vi "I2.vi"() -> ()   [LabVIEW 2020]
uses:
  <vilib>/Analysis/Matrix/Datatypes/RealMatrix.ctl
  <vilib>/Platform/TimedLoop/XDataNode/timing_clust.ctl
  <vilib>/Platform/TimedLoop/XDataNode/nitl_modes.ctl
  <vilib>/Platform/TimedLoop/XDataNode/wakeup.ctl
  <vilib>/Analysis/baseanly.llb/Real Dot Product.vi
  <vilib>/MakerHub/LINX/Public/Peripherals/PWM/PWM Set Duty Cycle 1 Chan.vi
  <vilib>/MakerHub/LINX/Public/Peripherals/Analog/Analog Read 1 Chan.vi
  <vilib>/MakerHub/LINX/Public/Peripherals/Analog/Analog Read N Chans.vi
  <vilib>/MakerHub/LINX/Private/Local IO/LinxAnalogRead.vi
  <vilib>/MakerHub/LINX/Public/Utilities/Check Channel.vi
  <vilib>/MakerHub/LINX/Public/Utilities/Open Serial.vi
  <vilib>/MakerHub/LINX/Public/Peripherals/PWM/PWM Set Duty Cycle N Chans.vi
  <vilib>/MakerHub/LINX/Private/Utilties/Generate Error.vi
  <vilib>/Analysis/polynomials.llb/Create Polynomial From Roots (CDB).vi
  <vilib>/platform/TimedLoop/XDataNode/XDataNode.xnode
  <vilib>/MakerHub/LINX/LMH-LINX.lvlib
  <vilib>/Platform/TimedLoop/XDataNode/XDNodeRunTimeDep.lvlib
  <vilib>/Analysis/NI_AALPro.lvlib
  <vilib>/Analysis/NI_AALBase.lvlib
  <vilib>/Analysis/Matrix/NI_Matrix.lvlib
panel:
  in  "file path (use dialog)":path
  out "corriente":dbl
  out "A":T1
  out "Regresor":dbl[](array[numeric])
  out "Pd(Z)":dbl[](array[numeric])
  out "p/q":dbl[](array[numeric]) format="%.4f"
  out "Theta":dbl[](array[numeric])
  in  "Parametros":T2={"Lambda"=0.987, "Alfa"=10000.0, "nb"=2, "d"=2, "na"=2, "b0? "=FALSE}
  in  "Pnd":cdb[](array[numeric])=[0.1+0.0i, 0.1+0.0i, 0.1+0.0i, 0.1+0.0i]
  in  "ts(s)":dbl=100.0
  in  "Tm":dbl=1.0
  in  "Mp(%)":dbl=5.0
  in  "Setpoint":dbl
  out "u(k)":dbl
  out "Temperatura":dbl
  out "x/y":dbl
  in  "stop":bool
  in  "Serial Port":refnum<visa-resource-name>="N/A"
  out "?":cluster{"Temperatura":dbl, dbl, "u(k)":dbl}(graph)
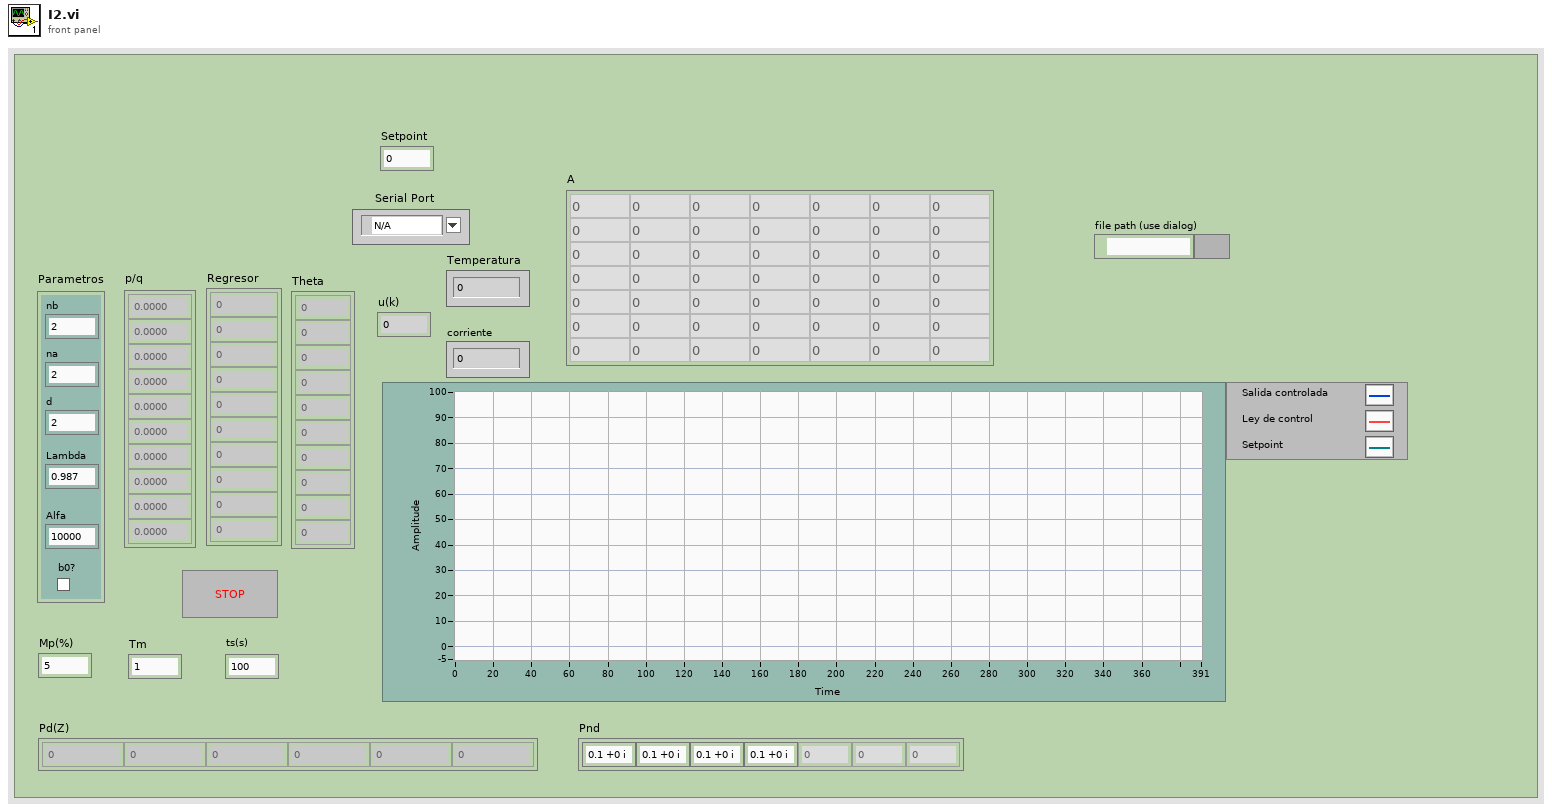
[diagram p1: front panel]
types:
  T1 = typedef "NI_Matrix.lvlib/RealMatrix.ctl" = dbl[][]
  T2 = cluster{"Lambda":dbl, "Alfa":dbl, "nb":u8, "d":u8, "na":u8, "b0? ":bool}
  T3 = enum16{"open", "replace", "create", "open or create", "replace or create", "replace or create with confirmation"}
  T4 = typedef "LMH-LINX.lvlib/LINX Ref.ctl" = cluster{"IO":T5, "Interface":T6, "LINX Device Config":T7}
  T5 = typedef "LMH-LINX.lvlib/Platform.ctl" = enum16{"Remote", "Local"}
  T6 = typedef "LMH-LINX.lvlib/Interface.ctl" = enum16{"Serial", "TCP"}
  T7 = typedef "LMH-LINX.lvlib/Device.lvlib/LINX Device Config.ctl" = cluster{"Interface":T6, "COM Port":refnum<visa-resource-name>, "TCP Configuration":T8, "Device Family":u8, "Device ID":u8, "Device Name":string, "TCP Ref":refnum<k5>, "Channels":T9}
  T8 = typedef "LMH-LINX.lvlib/Device.lvlib/TCP Config.ctl" = cluster{"IP Address":string, "Port":u16}
  T9 = typedef "LMH-LINX.lvlib/Channels.ctl" = cluster{"DI":u8[], "DO":u8[], "AI":u8[], "AO":u8[], "PWM":u8[], "QE":u8[], "UART":u8[], "I2C 2":u8[], "SPI":u8[], "CAN":u8[], "Servo":u8[], "AI Ref (V)":dbl, "AI Resolution (Bits)":u8, "AO Ref (V)":dbl, "AO Resolution (Bits)":u8}
  T10 = typedef "XDNodeRunTimeDep.lvlib/timing_clust.ctl" = cluster{"Expected End [f-1]":u64, "Actual End [f-1]":u64, "Finished Late? [f-1]":bool, "Expected End [i-1]":u64, "Actual End [i-1]":u64, "Finished Late? [i-1]":bool, "Expected Start [i]":u64, "Actual Start [i]":u64, "Expected Start [f]":u64, "Actual Start [f]":u64, "Source Name":string, "Structure Name":string, "Period":i64, "Deadline":i64, "Offset":i64, "Start":i64, "Priority":i32, "Timeout":i32, "Mode":T11, "Wakeup Reason":T12, "Error":errorcluster, "Source Type":string, "Secondary Source Type":string, "Global End Time":u64, "Global Start Time":u64, "Frame Duration":u64, "Iteration Duration":u64, "Assigned CPU":i32, "I/O Scan Engine Mode":u32}
  T11 = typedef "XDNodeRunTimeDep.lvlib/nitl_modes.ctl" = enum32{"No Change", "Process missed periods, maintain original phase", "Discard missed periods, maintain original phase", "Process missed periods, ignore original phase", "Discard missed periods, ignore original phase"}
  T12 = typedef "XDNodeRunTimeDep.lvlib/wakeup.ctl" = enum32{"Normal", "Aborted", "Asynchronous wakeup", "Timing source error", "Timed loop error", "Timeout"}
  T13 = cluster{"Temperatura":dbl, "u(k)":dbl, "Setpoint":dbl}
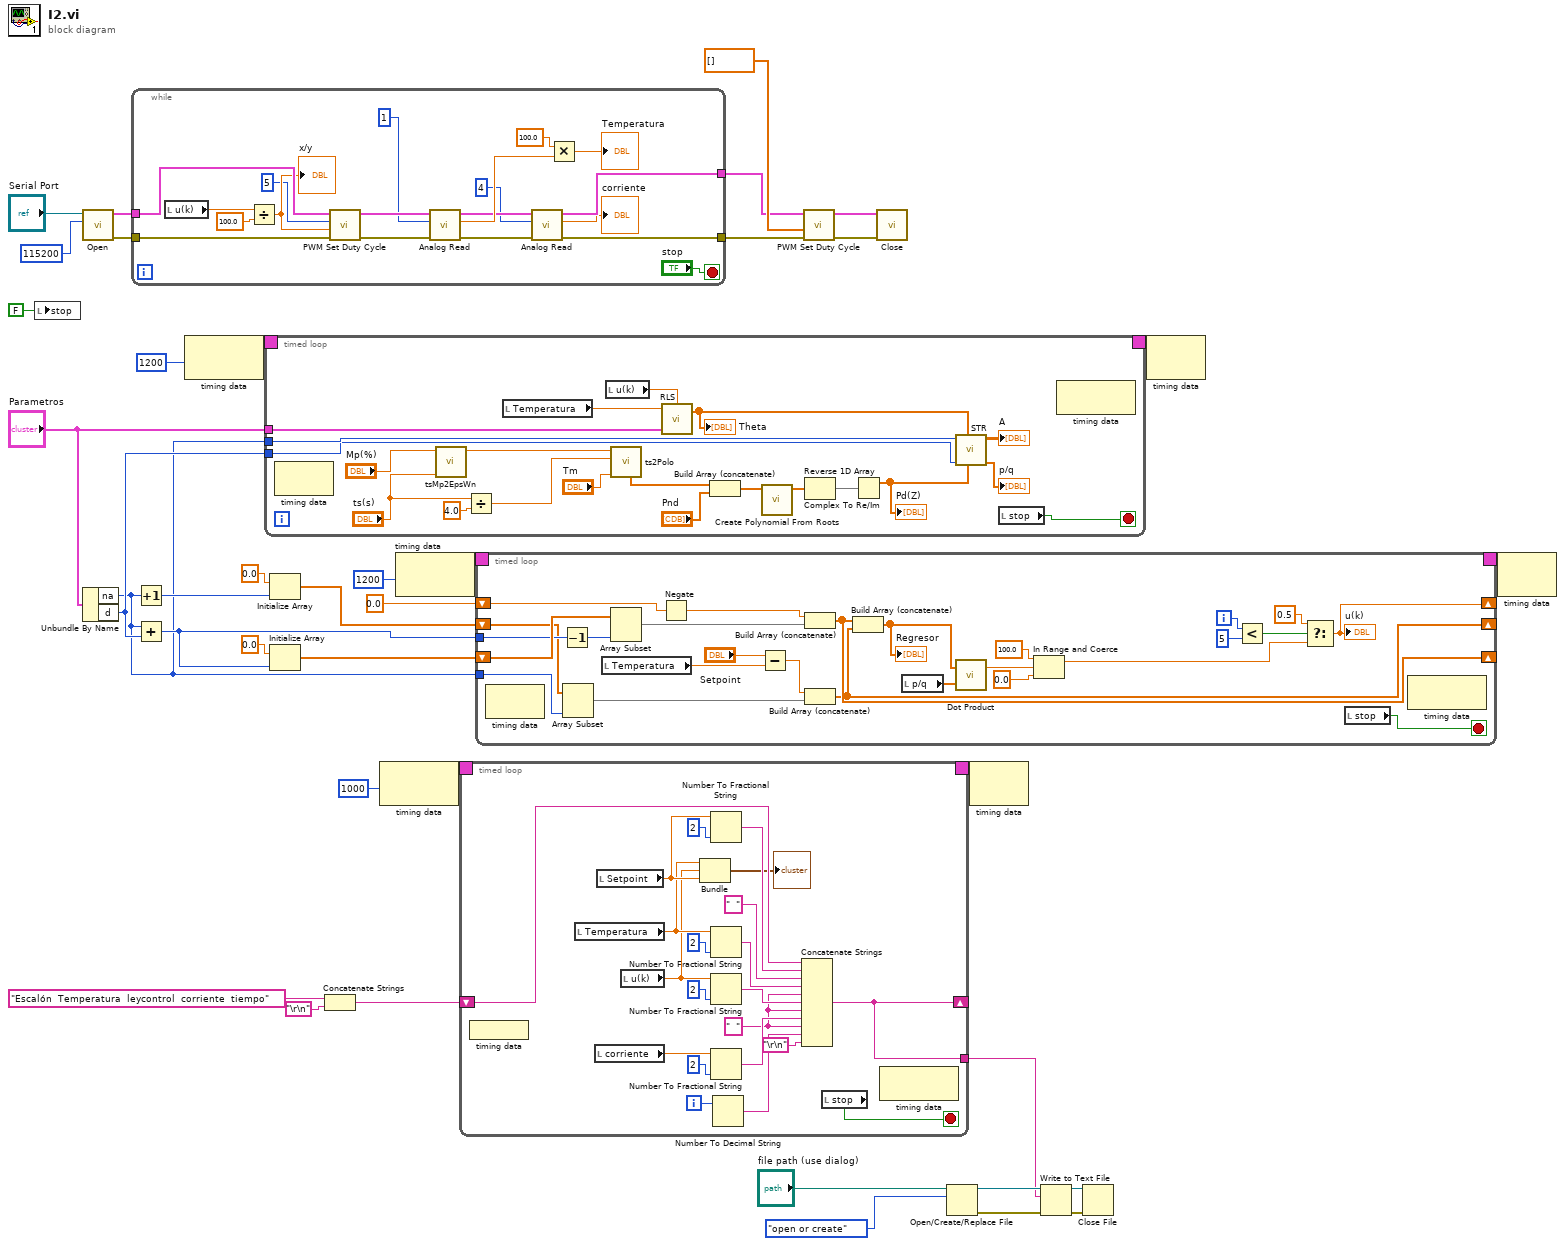
[diagram p0: block diagram]
diagram:
  n1 = local write "stop"(FALSE ("stop")) -> ()
  n2 = call-poly <vilib>:"Open.vi"("Baud Rate Override"=u32 115200, "Serial Port"="Serial Port") -> ("Error Out"=w31:errorcluster, "LINX Resource"=w32:T4)  [unwired: 7 in, 1 out]
  n3 = Unbundle By Name("Parametros") -> ("na"=w15:u8, "d"=w19:u8)
  n4 = while {
    tunnel: w32 -> [w58]
    tunnel: [w43] -> w34
    tunnel: w31 -> [w56]
    tunnel: [w42] -> w35
    stop <- "stop" stop-if-true
    n5 = local read "u(k)"() -> (w47:dbl)
    n6 = Divide(x=w47, y=100.0) -> (x/y=w51:dbl)
    "x/y" <- w51
    n7 = call-poly <vilib>:"PWM Set Duty Cycle.vi"("Error In"=w56, "Duty Cycle (0-1)"=w51, "PWM Channel"=u8 5, "LINX Resource"=w58) -> ("Error Out"=w55:errorcluster, "LINX Resource"=w57:T4)  [unwired: 6 in]
    n8 = call-poly <vilib>:"Analog Read.vi"("Error In"=w55, "Analog Channel"=u8 1, "LINX Resource"=w57) -> ("Error Out"=w44:errorcluster, "Voltage"=w53:dbl, "LINX Resource"=w45:T4)  [unwired: 5 in, 1 out]
    n9 = call-poly <vilib>:"Analog Read.vi"("Error In"=w44, "Analog Channel"=u8 4, "LINX Resource"=w45) -> ("Error Out"=w42:errorcluster, "Voltage"=→"corriente":dbl, "LINX Resource"=w43:T4)  [unwired: 5 in, 1 out]
    n10 = Multiply(x=100.0, y=w53) -> (x*y=→"Temperatura":dbl)
  }
  n11 = Increment(x=w15) -> (x+1=w21:u8)
  n12 = Add(x=w15, y=w19) -> (x+y=w16:u8)
  n13 = node-c288(i64 1200 ("Period")) -> (w29:T10)
  n14 = timed-loop {
    timing: w29 -> [_]
    timing-out: [_] -> w28
    tunnel: "Parametros" -> [w68]
    tunnel: w15 -> [w61]
    tunnel: w19 -> [w60]
    stop <- w62 stop-if-true
    n15 = node-c288() -> ()  [unwired: 1 in, 1 out]
    n16 = call "tsMp2EpsWn.vi"("ts(s)"="ts(s)", "Mp(%)"="Mp(%)") -> ("Epsilon"=w69:dbl)  [unwired: 8 in, 1 out]
    n17 = Divide(x="ts(s)", y=4.0) -> (x/y=w76:dbl)
    n18 = local read "Temperatura"() -> (w66:dbl)
    n19 = local read "u(k)"() -> (w67:dbl)
    n20 = call "ts2Polo.vi"("Tm"="Tm", "Tao"=w76, "Epsilon"=w69) -> ("Polos (Z1,Z2)"=w75:cdb[])  [unwired: 6 in, 2 out]
    n21 = call "RLS.vi"("u(k)"=w67, "Parametros"=w68, "y(k)"=w66) -> ("Theta"=w65:dbl[])  [unwired: 1 in, 1 out]
    "Theta" <- w65
    n22 = Build Array (concatenate)(w75, "Pnd") -> (w73:cdb[])
    n23 = call-poly <vilib>:"Create Polynomial From Roots.vi"("Roots"=w73) -> ("P(x)"=w72:cdb[])  [unwired: 9 in, 1 out]
    n24 = Reverse 1D Array(array=w72) -> (reversed array=w71:cdb[])
    n25 = Complex To Re/Im(x + iy=w71) -> (x=w64:dbl[])  [unwired: 1 out]
    "Pd(Z)" <- w64
    n26 = call "STR.vi"("Pd(z)"=w64, "Theta in"=w65, "d"=w60, "m"=w61) -> ("p/q"=→"p/q":dbl[], "A"=→"A":T1)  [unwired: 6 in]
    n27 = local read "stop"() -> (w62:bool)
    n28 = node-c288() -> ()  [unwired: 1 in, 1 out]
  }
  n29 = Initialize Array(0.0 ("element"), w21) -> (w17:dbl[])
  n30 = Initialize Array(0.0 ("element"), w16) -> (w18:dbl[])
  n31 = Concatenate Strings("Escalón  Temperatura  leycontrol  corriente  tiempo" ("string"), "\r\n") -> (w13:string)
  n32 = node-c288(i64 1000 ("Period")) -> (w3:T10)
  n33 = node-c288(i64 1200 ("Period")) -> (w26:T10)
  n34 = timed-loop {
    shift-right: [w96] -> _
    shift-left: w13 -> [w97]
    tunnel: [w96] -> w6
    timing: w3 -> [_]
    timing-out: [_] -> w2
    i -> [w101]
    stop <- w92 stop-if-true
    w89 = "  " ("string")
    n35 = node-c288() -> ()  [unwired: 1 in]
    n36 = local read "Temperatura"() -> (w83:dbl)
    n37 = local read "corriente"() -> (w86:dbl)
    n38 = local read "Setpoint"() -> (w84:dbl)
    n39 = local read "u(k)"() -> (w82:dbl)
    n40 = Bundle("Temperatura"=w83, "u(k)"=w82, "Setpoint"=w84) -> (→"?":T13)  [unwired: 1 in]
    n41 = Number To Fractional String(number=w84, precision (6)=i16 2) -> (F-format string=w100:string)  [unwired: 2 in]
    n42 = Number To Fractional String(number=w83, precision (6)=i16 2) -> (F-format string=w99:string)  [unwired: 2 in]
    n43 = Number To Fractional String(number=w82, precision (6)=i16 2) -> (F-format string=w90:string)  [unwired: 2 in]
    n44 = Number To Fractional String(number=w86, precision (6)=i16 2) -> (F-format string=w93:string)  [unwired: 2 in]
    n45 = Number To Decimal String(number=w101) -> (decimal integer string=w88:string)  [unwired: 1 in]
    n46 = Concatenate Strings(w97, w100, "  " ("string"), w99, w89, w90, w89, w93, w89, w88, "\r\n") -> (w96:string)
    n47 = local read "stop"() -> (w92:bool)
    n48 = node-c288() -> ()  [unwired: 1 in, 1 out]
  }
  n49 = timed-loop {
    timing: w26 -> [_]
    timing-out: [_] -> w25
    shift-right: [w121] -> _
    shift-left: w18 -> [w129]
    shift-right: [w120] -> _
    shift-left: w17 -> [w126]
    tunnel: w16 -> [w128]
    tunnel: w15 -> [w127]
    shift-right: [w105] -> _
    shift-left: 0.0 ("upper limit") -> [w108]
    i -> [w113]
    stop <- w109 stop-if-true
    n50 = node-c288() -> ()  [unwired: 1 in, 1 out]
    n51 = Decrement(x=w128) -> (x-1=w130:u8)
    n52 = Array Subset(array=w126, length=w127) -> (w123:dbl[])  [unwired: 1 in]
    n53 = local read "Temperatura"() -> (w125:dbl)
    n54 = Array Subset(array=w129, length=w130) -> (w122:dbl[])  [unwired: 1 in]
    n55 = Negate(x=w108) -> (-x=w107:dbl)
    n56 = Subtract(x="Setpoint", y=w125) -> (x-y=w124:dbl)
    n57 = Build Array (concatenate)(w107, w122) -> (w121:dbl[])
    n58 = Build Array (concatenate)(w124, w123) -> (w120:dbl[])
    n59 = Build Array (concatenate)(w121, w120) -> (w110:dbl[])
    "Regresor" <- w110
    n60 = local read "p/q"() -> (w119:dbl[])
    n61 = call-poly <vilib>:"Dot Product.vi"("Y Vector"=w119, "X Vector"=w110) -> ("X * Y"=w118:dbl)  [unwired: 1 out]
    n62 = In Range and Coerce(upper limit=100.0, x=w118, lower limit=0.0) -> (coerced(x)=w115:dbl)  [unwired: 1 out]
    n63 = Less?(x=w113, y=5) -> (x < y?=w111:bool)
    n64 = Select(t=0.5, s=w111, f=w115) -> (s? t:f=w105:dbl)
    "u(k)" <- w105
    n65 = local read "stop"() -> (w109:bool)
    n66 = node-c288() -> ()  [unwired: 1 in, 1 out]
  }
  n67 = call-poly <vilib>:"PWM Set Duty Cycle.vi"("Error In"=w35, "Duty Cycles"=dbl[] [], "LINX Resource"=w34) -> ("Error Out"=w37:errorcluster, "LINX Resource"=w36:T4)  [unwired: 7 in]
  n68 = call <vilib>:"Close.vi"("Error In"=w37, "LINX Resource"=w36) -> ()  [unwired: 9 in, 1 out]
  n69 = Open/Create/Replace File(file path (use dialog)="file path (use dialog)", operation (0:open)=T3."open or create") -> (refnum out=w7:refnum<file>, error out=w8:errorcluster)  [unwired: 4 in, 1 out]
  n70 = node-c288(w2) -> ()  [unwired: 1 out]
  n71 = Write to Text File(file (use dialog)=w7, text=w6, error in=w8) -> (refnum out=w4:refnum<file>, error out=w5:errorcluster)  [unwired: 1 in, 1 out]
  n72 = Close File(refnum=w4, error in=w5) -> ()  [unwired: 2 out]
  n73 = node-c288(w28) -> ()  [unwired: 1 out]
  n74 = node-c288(w25) -> ()  [unwired: 1 out]
